vi "Busy Icon & Message Storage.vi"(4 "Get(F)/Set Message":bool, 6 "Get(F)/Set Busy Icon":bool, 8 "Error In":errorcluster, 10 "Message String":string, 11 "Busy Icon Status (F = busy)":bool) -> (0 "Error Out":errorcluster, 2 "Message String":string, 3 "Busy Icon Status (F = busy)":bool)   [LabVIEW 2021, in "GUI.lvlib"]
uses:
  GUI.lvlib
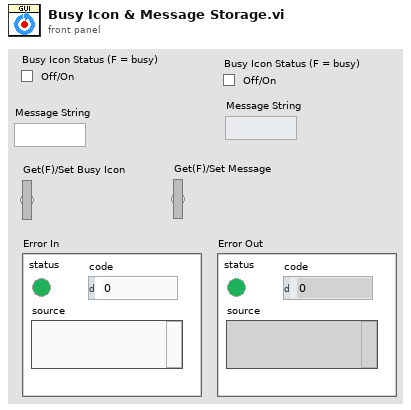
[diagram p1: front panel]
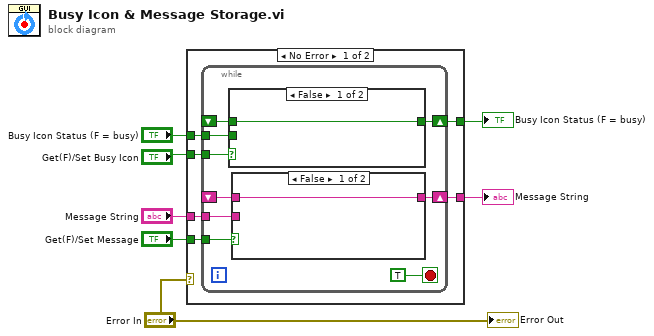
[diagram p0: block diagram]
diagram:
  n1 = case shown="No Error" "Error In" {
    tunnel: "Get(F)/Set Busy Icon" -> [w13 _]
    tunnel: "Busy Icon Status (F = busy)" -> [w12 _]
    tunnel: [w11 _] -> w5
    tunnel: "Message String" -> [w10 _]
    tunnel: [w9 _] -> w3
    tunnel: "Get(F)/Set Message" -> [w8 _]
    frame No Error {
      n2 = while {
        tunnel: w13 -> [w21]
        shift-right: [w20] -> w11
        shift-left: _ -> [w18]
        shift-right: [w16] -> w9
        shift-left: _ -> [w14]
        tunnel: w12 -> [w19]
        tunnel: w10 -> [w15]
        tunnel: w8 -> [w17]
        stop <- TRUE stop-if-true
        n3 = case shown="False" w21 {
          tunnel: [w25 w26] -> w20
          tunnel: w19 -> [_ w26]
          tunnel: w18 -> [w25 _]
          frame False {
          }
          frame True {
          }
        }
        n4 = case shown="False" w17 {
          tunnel: [w23 w24] -> w16
          tunnel: w15 -> [_ w24]
          tunnel: w14 -> [w23 _]
          frame False {
          }
          frame True {
          }
        }
      }
    }
    frame Error {
    }
  }
  "Busy Icon Status (F = busy)" <- w5
  "Message String" <- w3
  "Error Out" <- "Error In"
